vi "Flywheel_Execute.vi"() -> ()   [LabVIEW 2019]
uses:
  Globals/Flywheel_Globals.vi
  <vilib>/Rock Robotics/WPI/ThirdParty/REV Robotics/SPARK MAX/Typedef/Spark MAX Control Type.ctl
  Globals/Sensor_Values.vi
panel:
  out "Spun-Up":bool
  out "Error":dbl
  in  "Acceptable_error":dbl=150.0
  in  "Ramp Rate Auto":sgl
  in  "Ramp Rate Manual":sgl=0.25
  in  "Max Speed":dbl=5100.0
  # "Click here to set min"
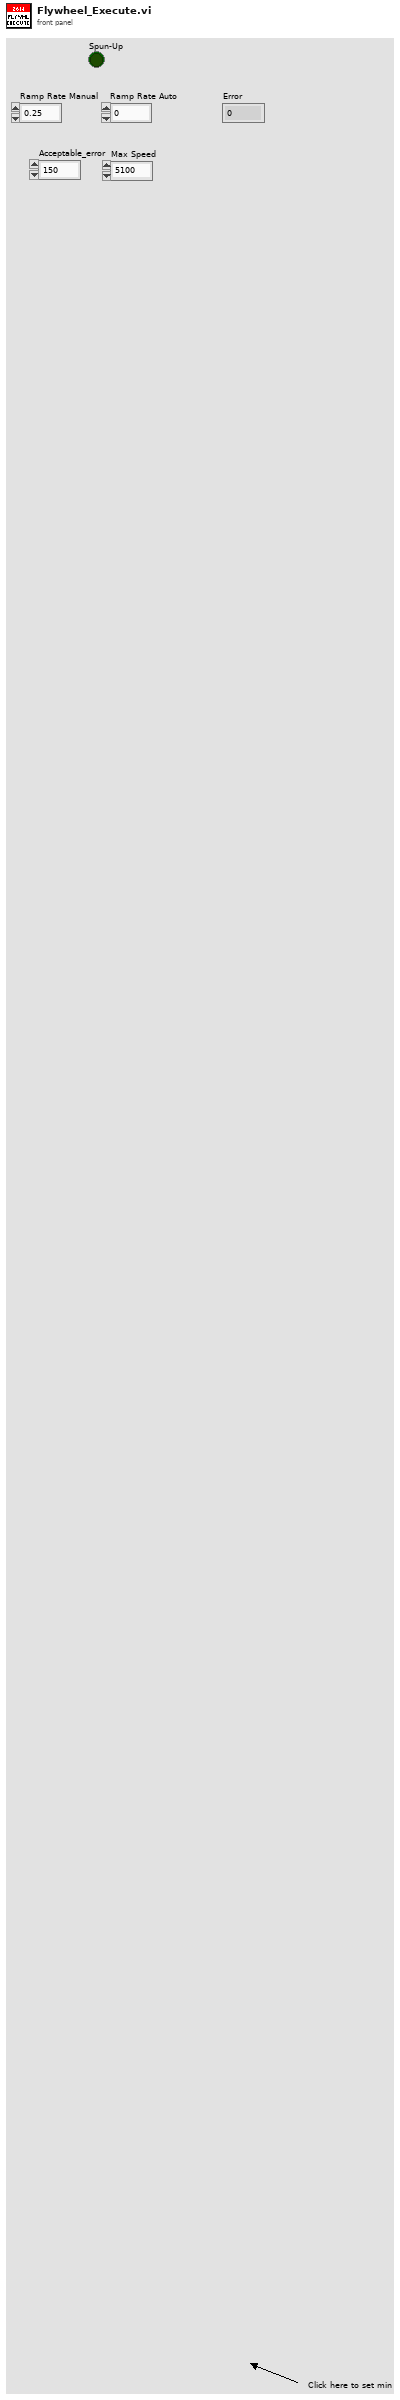
[diagram p1: front panel]
types:
  T1 = typedef "WPI_MotorControlDeviceRef.ctl" = cluster{"DeviceStatus":errorcluster, "Type":T2, "PWM":cluster{"PWM Channel":T3, "DeadBand":T4}, "CAN":cluster{"Device Number":u8, "SetOutput VI Ref":variant, "GetOutput VI Ref":variant, "Enable VI Ref":variant, "Disable VI Ref":variant, "Data":variant}, "Invert":bool, "DIO PWM":cluster{"PWM \"Enable\" Channel":T3, "DIOChannel":T5, "PWM Rate":dbl}}
  T2 = typedef "WPI_MotorControlType.ctl" = enum16{"PWM", "CAN", "DIO PWM"}
  T3 = typedef "FPGA_DIOPWMChannel.ctl" = enum8{"PWM 0", "PWM 1", "PWM 2", "PWM 3", "PWM 4", "PWM 5", "PWM 6", "PWM 7", "PWM 8", "PWM 9", "PWM MXP 0", "PWM MXP 1", "PWM MXP 2", "PWM MXP 3", "PWM MXP 4", "PWM MXP 5", "PWM MXP 6", "PWM MXP 7", "PWM MXP 8", "PWM MXP 9", "Invalid"}
  T4 = typedef "WPI_PWMDeadband.ctl" = cluster{"Name":string, "maxPositivePwm":i32, "minPositivePwm":i32, "centerPwm":i32, "maxNegativePwm":i32, "minNegativePwm":i32, "angularRange":u16}
  T5 = typedef "FPGA_DIOChannel.ctl" = enum8{"DIO 0", "DIO 1", "DIO 2", "DIO 3", "DIO 4", "DIO 5", "DIO 6", "DIO 7", "DIO 8", "DIO 9", "DIO MXP 0", "DIO MXP 1", "DIO MXP 2", "DIO MXP 3", "DIO MXP 4", "DIO MXP 5", "DIO MXP 6", "DIO MXP 7", "DIO MXP 8", "DIO MXP 9", "DIO MXP 10", "DIO MXP 11", "DIO MXP 12", "DIO MXP 13", "DIO MXP 14", "DIO MXP 15", "SPI Port CS1", "SPI Port CS2", "SPI Port CS3", "SPI Port MISO", "SPI Port MOSI", "Invalid"}
  T6 = typedef "Spark MAX Control Type.ctl" = enum16{"Percent VBus", "Voltage", "Velocity", "Position", "Smart Motion", "Current", "Smart Velocity"}
  T7 = typedef "Flywheel_Cluster.ctl" = cluster{"Flywheel_Throttle":dbl, "Control_States":T8, "Auto_Speed":bool, "Flywheel_On":bool}
  T8 = typedef "Flywheel_States.ctl" = enum16{"No-Op", "Percent_Voltage", "Speed_Control_Manual", "Speed_Control_Auto"}
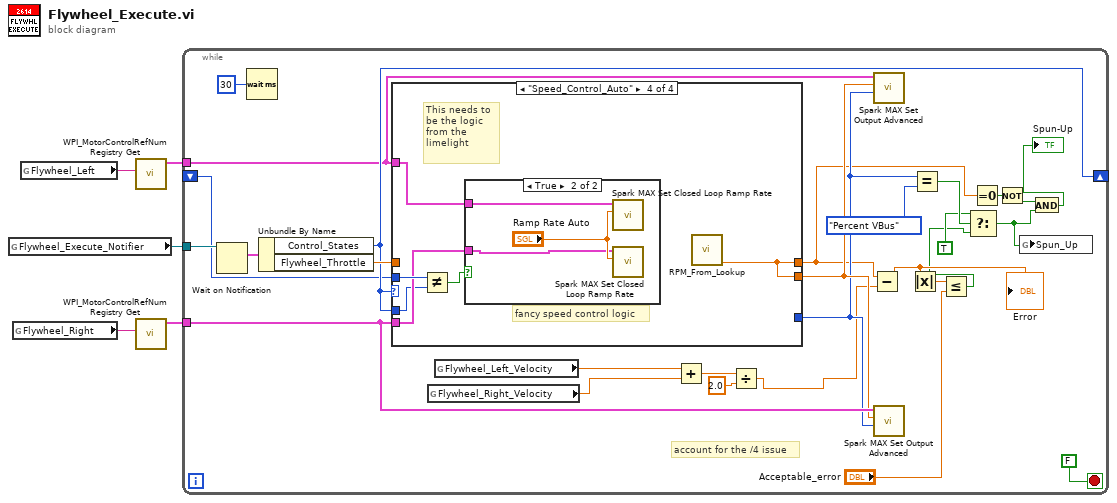
[diagram p0: block diagram]
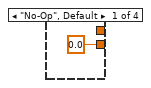
[diagram p2: hidden frame]
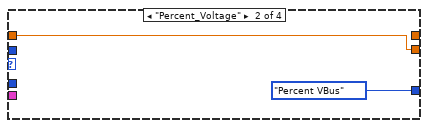
[diagram p3: hidden frame]
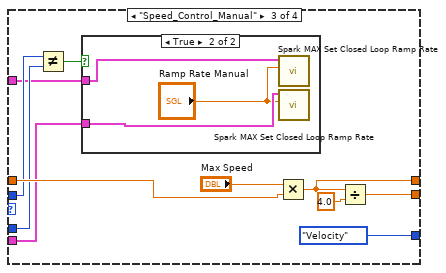
[diagram p4: hidden frame]
diagram:
  n1 = global read "Flywheel_Globals.vi" "Flywheel_Execute_Notifier"() -> (w5:refnum<notifier>)
  n2 = global read "Flywheel_Globals.vi" "Flywheel_Right"() -> (w4:string)
  n3 = global read "Flywheel_Globals.vi" "Flywheel_Left"() -> (w3:string)
  n4 = call <vilib>:"WPI_MotorControlRefNum Registry Get.vi"("refnum name"=w3) -> ("MotorControlDevRef"=w2:T1)  [unwired: 9 in, 1 out]
  n5 = call <vilib>:"WPI_MotorControlRefNum Registry Get.vi"("refnum name"=w4) -> ("MotorControlDevRef"=w1:T1)  [unwired: 9 in, 1 out]
  n6 = while {
    tunnel: w5 -> [w32]
    tunnel: w2 -> [w26]
    tunnel: w1 -> [w25]
    shift-right: [w28] -> _
    shift-left: _ -> [w27]
    stop <- FALSE stop-if-true
    # "account for the /4 issue"
    n7 = Wait on Notification(notifier=w32) -> (notification=w31:T7)  [unwired: 3 in, 3 out]
    n8 = Wait (ms)(milliseconds to wait=u32 30) -> ()  [unwired: 1 out]
    n9 = Unbundle By Name(w31) -> ("Control_States"=w28:T8, "Flywheel_Throttle"=w30:dbl)
    n10 = case shown="\"Speed_Control_Auto\"" w28 {
      tunnel: [0.0 ("Flywheel_Throttle") w36 w38 w51] -> w20
      tunnel: w30 -> [_ w36 w45 _]
      tunnel: [_ Spark_MAX_Control_Type."Percent VBus" ("Control Mode") Spark_MAX_Control_Type."Velocity" ("Control Mode") _] -> w16
      tunnel: w28 -> [_ _ w44 w52]
      tunnel: w27 -> [_ _ w43 w55]
      tunnel: w26 -> [_ _ w41 w54]
      tunnel: w25 -> [_ _ w40 w53]
      tunnel: [_ _ w37 w51] -> w8
      frame "No-Op", Default {
      }
      frame "Percent_Voltage" {
      }
      frame "Speed_Control_Manual" {
        n11 = Not Equal?(x=w43, y=w44) -> (x != y?=w42:bool)
        n12 = case shown="True" w42 {
          tunnel: w41 -> [_ w50]
          tunnel: w40 -> [_ w49]
          frame False {
          }
          frame True {
            n13 = call <vilib>:"Spark MAX Set Closed Loop Ramp Rate.vi"("Seconds from neutral to full (0)"="Ramp Rate Manual", "MotorControlDeviceRef in"=w50) -> ()  [unwired: 8 in, 2 out]
            n14 = call <vilib>:"Spark MAX Set Closed Loop Ramp Rate.vi"("Seconds from neutral to full (0)"="Ramp Rate Manual", "MotorControlDeviceRef in"=w49) -> ()  [unwired: 8 in, 2 out]
          }
        }
        n15 = Multiply(x="Max Speed", y=w45) -> (x*y=w37:dbl)
        n16 = Divide(x=w37, y=4.0) -> (x/y=w38:dbl)
      }
      frame "Speed_Control_Auto" {
        # "This needs to \nbe the logic \nfrom the \nlimelight"
        # "fancy speed control logic"
        n17 = Not Equal?(x=w55, y=w52) -> (x != y?=w56:bool)
        n18 = case shown="True" w56 {
          tunnel: w54 -> [_ w58]
          tunnel: w53 -> [_ w57]
          frame False {
          }
          frame True {
            n19 = call <vilib>:"Spark MAX Set Closed Loop Ramp Rate.vi"("Seconds from neutral to full (0)"="Ramp Rate Auto", "MotorControlDeviceRef in"=w58) -> ()  [unwired: 8 in, 2 out]
            n20 = call <vilib>:"Spark MAX Set Closed Loop Ramp Rate.vi"("Seconds from neutral to full (0)"="Ramp Rate Auto", "MotorControlDeviceRef in"=w57) -> ()  [unwired: 8 in, 2 out]
          }
        }
        n21 = call "RPM_From_Lookup.vi"() -> ("RPM output"=w51:dbl)  [unwired: 8 in, 3 out]
      }
    }
    n22 = global read "Sensor_Values.vi" "Flywheel_Right_Velocity"() -> (w23:dbl)
    n23 = global read "Sensor_Values.vi" "Flywheel_Left_Velocity"() -> (w24:dbl)
    n24 = Add(x=w24, y=w23) -> (x+y=w22:dbl)
    n25 = Divide(x=w22, y=2.0) -> (x/y=w13:dbl)
    n26 = Subtract(x=w8, y=w13) -> (x-y=w19:dbl)
    "Error" <- w19
    n27 = call <vilib>:"Spark MAX Set Output Advanced.vi"("Control Mode"=w16, "Setpoint"=w20, "MotorControlDevRef"=w26) -> ()  [unwired: 7 in, 2 out]
    n28 = call <vilib>:"Spark MAX Set Output Advanced.vi"("Control Mode"=w16, "Setpoint"=w20, "MotorControlDevRef"=w25) -> ()  [unwired: 7 in, 2 out]
    n29 = Absolute Value(x=w19) -> (abs(x)=w18:dbl)
    n30 = Equal?(x=w16, y=Spark_MAX_Control_Type."Percent VBus") -> (x = y?=w14:bool)
    n31 = Less Or Equal?(x=w18, y="Acceptable_error") -> (x <= y?=w11:bool)
    n32 = Select(t=TRUE, s=w14, f=w11) -> (s? t:f=w10:bool)
    n33 = Equal To 0?(x=w8) -> (x = 0?=w9:bool)
    n34 = Not(x=w9) -> (.not. x?=w6:bool)
    n35 = global write "Flywheel_Globals.vi" "Spun_Up"(w10) -> ()
    n36 = And(x=w6, y=w10) -> (x .and. y?=→"Spun-Up":bool)
  }
